vi "Driver - DTACQ - Download Continuous Data Block (Multiplexed - Signed 32 Bit).vi"(8 "error in":errorcluster, 9 "Number of Samples":i32, 10 "Number of Channels":i32, 11 "DTACQ Connection Data In":T1={"Description"="", "Address"="", "Port"=0, "timeout (ms)"=5000, "Termination Character"="\n", "TCP Connection Reference"=refnum, "Open Connection"=FALSE}) -> (0 "error out":errorcluster, 1 "Data Received":bool, 2 "Data":i32[][](array[numeric]), 3 "DTACQ Connection Data Out":T1={"Description"="", "Address"="", "Port"=0, "timeout (ms)"=5000, "Termination Character"="\n", "TCP Connection Reference"=refnum, "Open Connection"=FALSE})   [LabVIEW 2017, in "Communications Library.lvlib"]
doc: "Downloads multiplexed data from the DTACQ device, in 32 bit integer format, and reformats the data into a 2D array."
uses:
  Communications Library.lvlib
  Typedefs/DTACQ Connection Data--Cluster.ctl
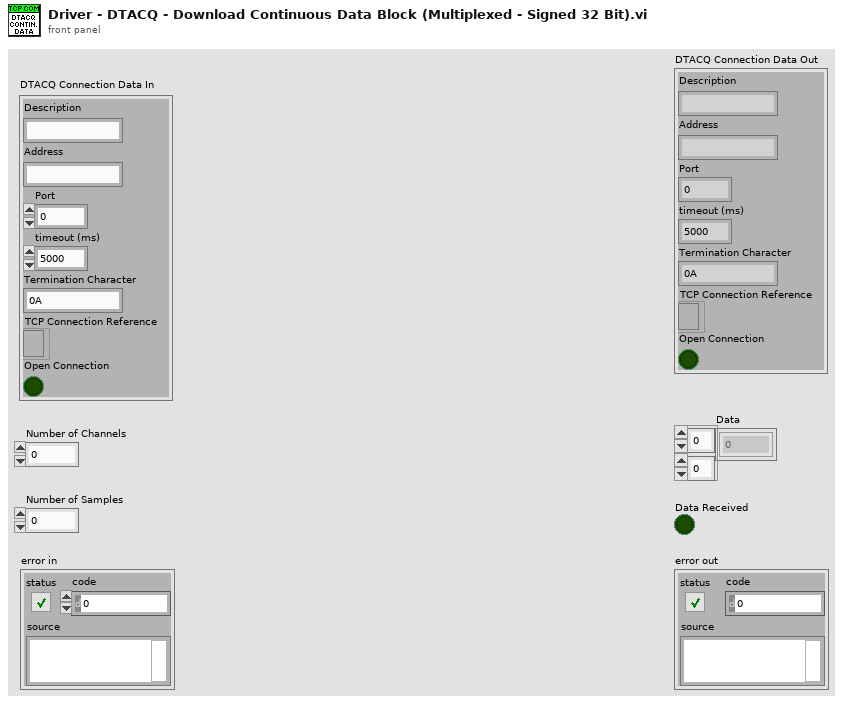
[diagram p1: front panel]
types:
  T1 = typedef "Communications Library.lvlib/DTACQ Connection Data--Cluster.ctl" = cluster{"Description":string, "Address":string, "Port":u16, "timeout (ms)":i32, "Termination Character":string, "TCP Connection Reference":refnum<k5>, "Open Connection":bool}
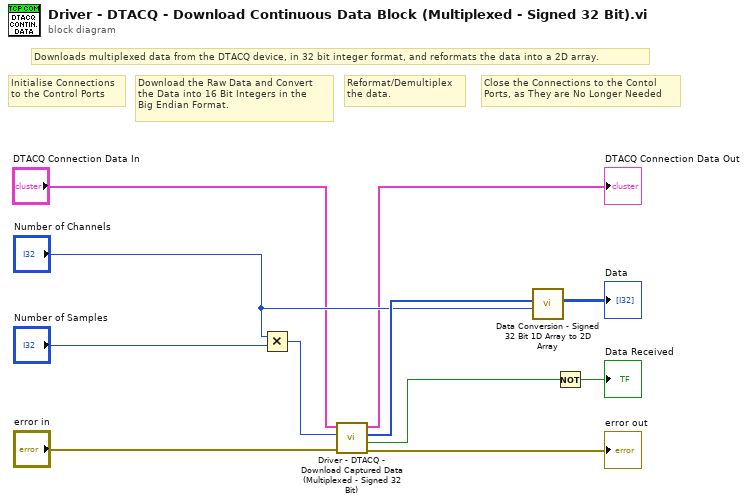
[diagram p0: block diagram]
diagram:
  # "Downloads multiplexed data from the DTACQ device, in 32 bit integer format, and reformats the data into a 2D array."
  # "Close the Connections to the Contol\nPorts, as They are No Longer Needed"
  # "Reformat/Demultiplex\nthe data."
  # "Download the Raw Data and Convert\nthe Data into 16 Bit Integers in the\nBig Endian Format."
  # "Initialise Connections\nto the Control Ports"
  n1 = Multiply(x="Number of Channels", y="Number of Samples") -> (x*y=w6:i32)
  n2 = call "Driver - DTACQ - Download Captured Data (Multiplexed - Signed 32 Bit).vi"("error in"="error in", "Samples"=w6, "DTACQ Connection Data In"="DTACQ Connection Data In") -> ("error out"=→"error out":errorcluster, "Timed Out"=w8:bool, "(Signed) 32 Bit Array"=w4:i32[], "DTACQ Connection Data Out"=→"DTACQ Connection Data Out":T1)  [unwired: 5 in]
  n3 = call "Data Conversion - Signed 32 Bit 1D Array to 2D Array.vi"("Channels"="Number of Channels", "1D Data (Multiplexed)"=w4) -> ("2D Data (De-Multiplexed)"=→"Data":i32[][])  [unwired: 9 in]
  n4 = Not(x=w8) -> (.not. x?=→"Data Received":bool)
